vi "Create.vi"(7 "VolatusAPI":refnum<class "VolatusAPI.lvclass">, 8 "error in (no error)":errorcluster, 10 "Channel":string) -> (0 "error out":errorcluster, 3 "Digital Command out":refnum<class "Digital Command.lvclass">)   [LabVIEW 2020, in "Volatus.lvlib" / "Digital Command.lvclass"]
uses:
  Digital Command.lvclass
  Digital Command.lvclass/Digital Command.ctl
  VolatusAPI/VolatusAPI.lvclass
  messages/CmdDigital/Data.ctl
  messages/CmdDigital/CmdDigital.lvlib
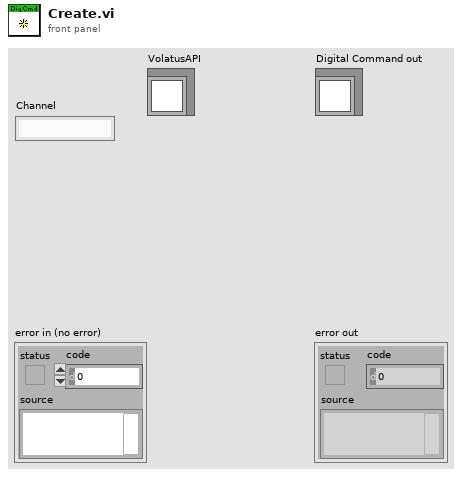
[diagram p1: front panel]
types:
  T1 = typedef "CmdDigital.lvlib/Data.ctl" = cluster{"channel":string, "value":bool}
  T2 = typedef "VectoConfig.lvlib/Channel Info.ctl" = cluster{"Name":string, "Group":string, "Owning Node":string, "Owning Task":string, "Resource":string}
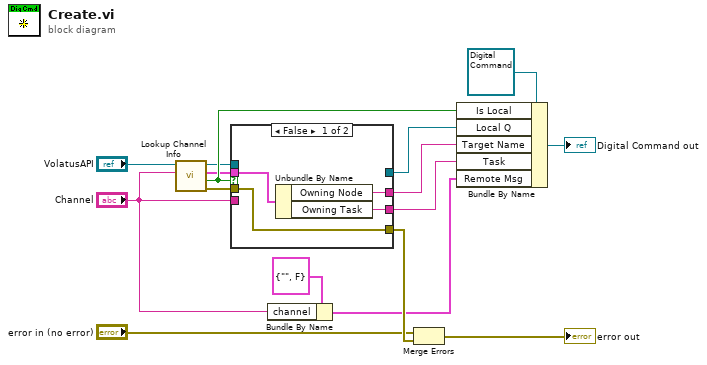
[diagram p0: block diagram]
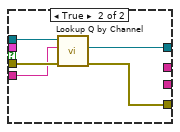
[diagram p2: hidden frame]
diagram:
  n1 = call "Lookup Channel Info.vi"("Channel Name"="Channel", "VolatusAPI in"="VolatusAPI") -> ("error out"=w2:errorcluster, "Local"=w11:bool, "Channel Info"=w5:T2, "VolatusAPI out"=w10:refnum<class "VolatusAPI.lvclass">)  [unwired: 6 in]
  n2 = case shown="False" w11 {
    tunnel: w10 -> [_ w24]
    tunnel: "Channel" -> [_ w23]
    tunnel: [_ w22] -> w8
    tunnel: w5 -> [w20 _]
    tunnel: [w19 _] -> w4
    tunnel: [w18 _] -> w3
    tunnel: w2 -> [w17 w25]
    tunnel: [w17 w21] -> w16
    frame False {
      n3 = Unbundle By Name(w20) -> ("Owning Node"=w19:string, "Owning Task"=w18:string)
    }
    frame True {
      n4 = call "Lookup Q by Channel.vi"("error in (no error)"=w25, "Channel Name"=w23, "VolatusAPI in"=w24) -> ("error out"=w21:errorcluster, "MessageQ"=w22:refnum<class "MessageQ.lvclass">)  [unwired: 6 in, 1 out]
    }
  }
  n5 = Bundle By Name(cluster=T1 {"channel"="", "value"=FALSE} ("Remote Msg"), "channel"="Channel") -> (w6:T1)
  n6 = Merge Errors("error in (no error)", w16) -> (→"error out":errorcluster)
  n7 = Bundle By Name(cluster=refnum<class "Digital Command.lvclass"> refnum ("Digital Command in"), "Is Local"=w11, "Local Q"=w8, "Target Name"=w4, "Task"=w3, "Remote Msg"=w6) -> (→"Digital Command out":refnum<class "Digital Command.lvclass">)
